vi "Empty Keyed Array.vi"() -> (1 "empty keyed array":T1)   [LabVIEW 2011]
uses:
  ITK EXT/utils/keyedarr.llb/Keyed Array.ctl
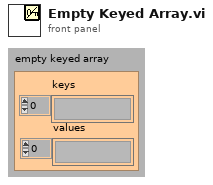
[diagram p1: front panel]
types:
  T1 = typedef "Keyed Array.ctl" = cluster{"keys":string[], "values":string[]}
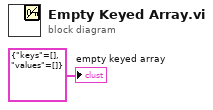
[diagram p0: block diagram]
diagram:
  "empty keyed array" <- T1 {"keys"=[], "values"=[]} ("array out")
